vi "Keithley6221Monitor.vi"   [LabVIEW 2016]
uses:
  Global/Global Variables/Data_Display_global.vi
  Instrument_Setup.vi
  <vilib>/ErrorRing/Error Ring.xnode
  Equipment/Keithley 622x/Keithley 622x.lvlib
types:
  T1 = typedef "Keithley 622x.lvlib/KE6221 -- Wave Sine Wave Params.ctl" = cluster{"Frequency (Hz)":T2, "Amplitude (A)":T3, "Offset (A)":T4, "Ranging Mode":T5, "Fixed Range":T6, "Playback Mode":T7, "Time (s)":T8, "Num Cycles":T9, "Phase\nMarker?":bool, "Phase Marker (deg)":T10, "Trig Link Line":T11}
  T2 = typedef "Keithley 622x.lvlib/KE6221 -- Wave Frequency.ctl" = dbl
  T3 = typedef "Keithley 622x.lvlib/KE6221 -- Wave Amplitude.ctl" = dbl
  T4 = typedef "Keithley 622x.lvlib/KE622x -- Current Level.ctl" = dbl
  T5 = typedef "Keithley 622x.lvlib/KE6221 -- Wave Ranging Mode.ctl" = enum16{"Best", "Fixed"}
  T6 = typedef "Keithley 622x.lvlib/KE622x -- Current Ranges.ctl" = enum16{"2nA", "20nA", "200nA", "2uA", "20uA", "200uA", "2mA", "20mA", "100mA"}
  T7 = typedef "Keithley 622x.lvlib/KE6221 -- Wave Playback Mode.ctl" = enum16{"Time", "Num Cycles"}
  T8 = typedef "Keithley 622x.lvlib/KE6221 -- Wave Playback Time.ctl" = dbl
  T9 = typedef "Keithley 622x.lvlib/KE6221 -- Wave Playback Num Cycles.ctl" = dbl
  T10 = typedef "Keithley 622x.lvlib/KE6221 -- Wave Phase Marker.ctl" = dbl
  T11 = typedef "Keithley 622x.lvlib/KE622x -- Trig Link Line.ctl" = enum16{"1", "2", "3", "4", "5", "6"}
  T12 = typedef "Keithley 622x.lvlib/KE622x -- On Off Control.ctl" = enum16{"Off", "On"}
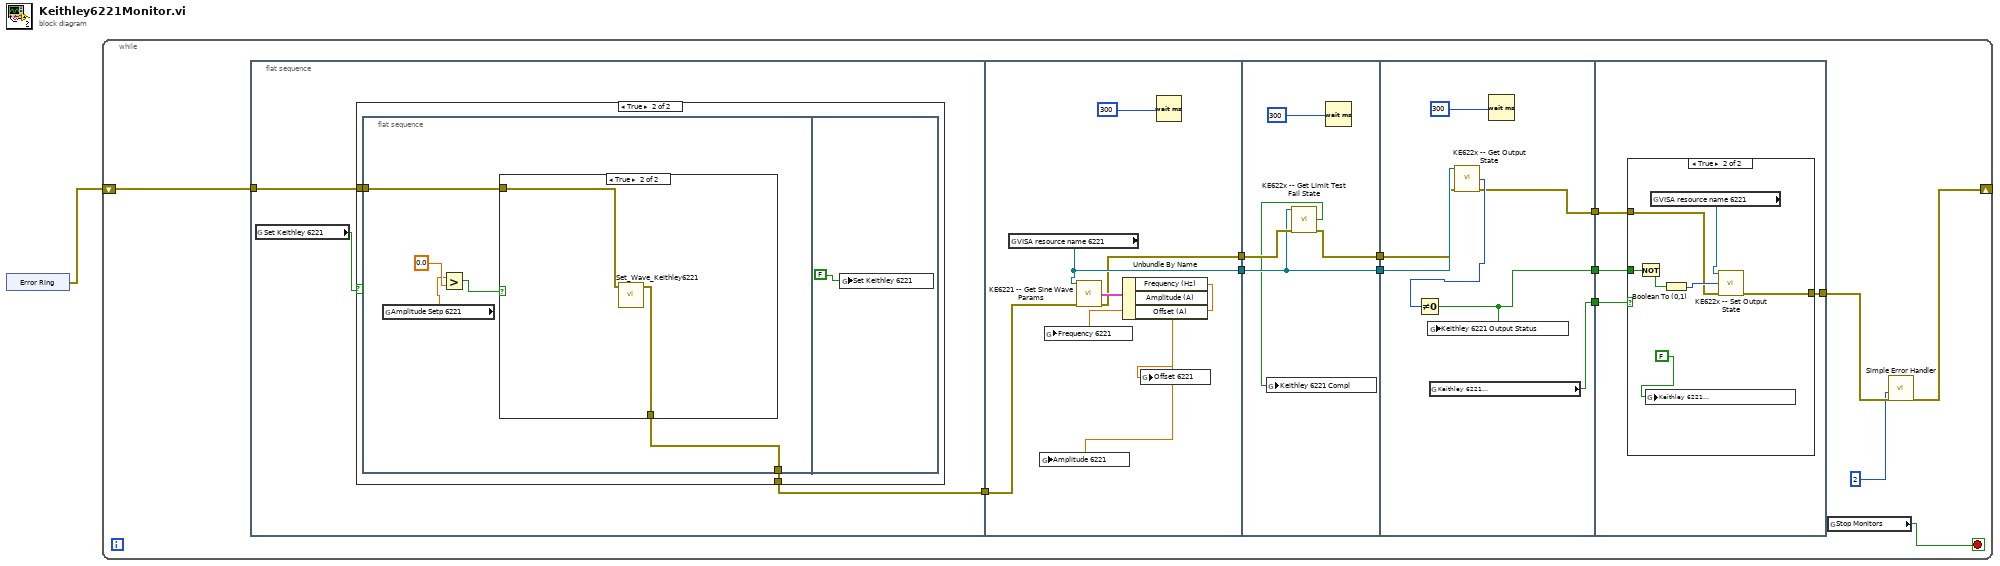
[diagram p0: block diagram]
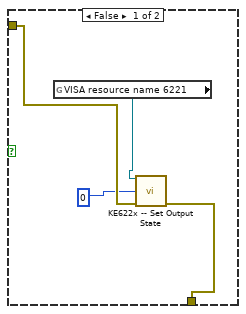
[diagram p3: hidden frame]
diagram:
  n1 = xnode "Error Ring"() -> ("error out"=w1:errorcluster)
  n2 = while {
    shift-right: [w3] -> _
    shift-left: w1 -> [w11]
    stop <- w14 stop-if-true
    n3 = flat-sequence {
      tunnel: w11 -> [w16]
      tunnel: [w15] -> w10
      tunnel: [w37] -> w8
      tunnel: w10 -> [w36]
      tunnel: [w35] -> w6
      tunnel: w8 -> [w42]
      tunnel: [w42] -> w7
      tunnel: w6 -> [w44]
      tunnel: [w43] -> w5
      tunnel: w7 -> [w51]
      tunnel: [w49] -> w13
      tunnel: [w48] -> w12
      tunnel: w5 -> [w47]
      tunnel: [w46] -> w9
      tunnel: w13 -> [w56]
      tunnel: w12 -> [w55]
      tunnel: w9 -> [w54]
      tunnel: [w53] -> w4
      frame #0 {
        n4 = global read "Data_Display_global.vi" "Set Keithley 6221"() -> (w17:bool)
        n5 = case shown="True" w17 {
          tunnel: w16 -> [w18 w20]
          tunnel: [w18 w19] -> w15
          frame False {
          }
          frame True {
            n6 = flat-sequence {
              tunnel: w20 -> [w22]
              tunnel: [w21] -> w19
              frame #0 {
                n7 = global read "Data_Display_global.vi" "Amplitude Setp 6221"() -> (w24:dbl)
                n8 = Greater?(x=w24, y=0.0) -> (0:w23:bool)
                n9 = case shown="True" w23 {
                  tunnel: w22 -> [w28 w31]
                  tunnel: [w27 w30] -> w21
                  frame False {
                    n10 = global read "Instrument_Setup.vi" "VISA resource name 6221"() -> (w29:refnum<visa-resource-name>)
                    n11 = call "KE622x -- Set Output State.vi"("Resource In"=w29, "Output State"=0, "error in (no error)"=w28) -> ("error out"=w27:errorcluster)  [unwired: 11 in, 1 out]
                  }
                  frame True {
                    n12 = call "Set_Wave_Keithley6221.vi"("Error in"=w31) -> ("Erro out"=w30:errorcluster)  [unwired: 8 in]
                  }
                }
              }
              frame #1 {
                n13 = global write "Data_Display_global.vi" "Set Keithley 6221"(FALSE) -> ()
              }
            }
          }
        }
      }
      frame #1 {
        n14 = global read "Instrument_Setup.vi" "VISA resource name 6221"() -> (w37:refnum<visa-resource-name>)
        n15 = call "KE6221 -- Get Sine Wave Params.vi"("Resource In"=w37, "error in (no error)"=w36) -> ("Sine Wave Params"=w40:T1, "error out"=w35:errorcluster)  [unwired: 11 in, 1 out]
        n16 = Unbundle By Name(w40) -> ("Frequency (Hz)"=w39:T2, "Amplitude (A)"=w34:T3, "Offset (A)"=w33:T4)
        n17 = global write "Data_Display_global.vi" "Amplitude 6221"(w34) -> ()
        n18 = global write "Data_Display_global.vi" "Frequency 6221"(w39) -> ()
        n19 = global write "Data_Display_global.vi" "Offset 6221"(w33) -> ()
        n20 = Wait (ms)(milliseconds to wait=300) -> ()  [unwired: 1 out]
      }
      frame #2 {
        n21 = call "KE622x -- Get Limit Test Fail State.vi"("Resource In"=w42, "error in (no error)"=w44) -> ("Limit Test Failed (Compliance)?"=w41:bool, "error out"=w43:errorcluster)  [unwired: 11 in, 1 out]
        n22 = global write "Data_Display_global.vi" "Keithley 6221 Compl"(w41) -> ()
        n23 = Wait (ms)(milliseconds to wait=300) -> ()  [unwired: 1 out]
      }
      frame #3 {
        n24 = global read "Data_Display_global.vi" "Keithley 6221\nOutput ON/OFF"() -> (w49:bool)
        n25 = call "KE622x -- Get Output State.vi"("Resource In"=w51, "error in (no error)"=w47) -> ("Output State"=w52:T12, "error out"=w46:errorcluster)  [unwired: 11 in, 1 out]
        n26 = Not Equal To 0?(x=w52) -> (x != 0?=w48:bool)
        n27 = global write "Data_Display_global.vi" "Keithley 6221 Output Status"(w48) -> ()
        n28 = Wait (ms)(milliseconds to wait=300) -> ()  [unwired: 1 out]
      }
      frame #4 {
        n29 = case shown="True" w56 {
          tunnel: w55 -> [_ w64]
          tunnel: w54 -> [w57 w60]
          tunnel: [w57 w59] -> w53
          frame False {
          }
          frame True {
            n30 = Not(x=w64) -> (.not. x?=w62:bool)
            n31 = global write "Data_Display_global.vi" "Keithley 6221\nOutput ON/OFF"(FALSE) -> ()
            n32 = global read "Instrument_Setup.vi" "VISA resource name 6221"() -> (w63:refnum<visa-resource-name>)
            n33 = Boolean To (0,1)(Boolean=w62) -> (0, 1=w61:i16)
            n34 = call "KE622x -- Set Output State.vi"("Resource In"=w63, "Output State"=w61, "error in (no error)"=w60) -> ("error out"=w59:errorcluster)  [unwired: 11 in, 1 out]
          }
        }
      }
    }
    n35 = global read "Data_Display_global.vi" "Stop Monitors"() -> (w14:bool)
    n36 = call <vilib>:"Simple Error Handler.vi"("type of dialog (OK msg:1)"=2, "error in (no error)"=w4) -> ("error out"=w3:errorcluster)  [unwired: 3 in, 4 out]
  }
